vi "stopMotion.vi"(8 "error in (no error)":errorcluster, 11 "Model in":refnum<class "Model.lvclass">) -> (0 "error out":errorcluster, 3 "Model out":refnum<class "Model.lvclass">)   [LabVIEW 2013, in "Model.lvclass"]
uses:
  Model.lvclass
  Model.lvclass/Model.ctl
  ApplicationElements/StepperMotor/StepperMotor.lvclass/StepperMotor.ctl
  ApplicationElements/StepperMotor/StepperMotor.lvclass
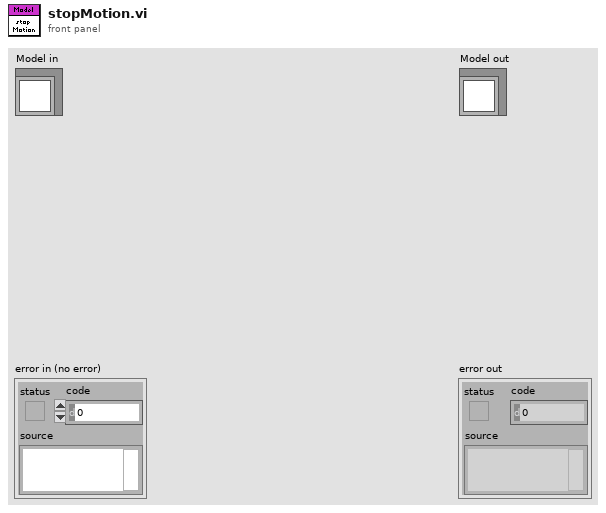
[diagram p1: front panel]
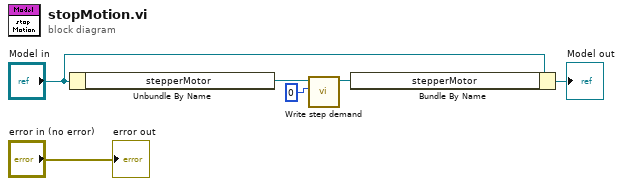
[diagram p0: block diagram]
diagram:
  n1 = Unbundle By Name("Model in") -> ("stepperMotor"=w5:refnum<class "StepperMotor.lvclass">)
  n2 = call "Write step demand.vi"("step demand"=i16 0, "StepperMotor in"=w5) -> ("StepperMotor out"=w4:refnum<class "StepperMotor.lvclass">)  [unwired: 9 in]
  n3 = Bundle By Name(cluster="Model in", "stepperMotor"=w4) -> (→"Model out":refnum<class "Model.lvclass">)
  "error out" <- "error in (no error)"
